vi "Save AO.vi"(8 "error in (no error)":errorcluster, 11 "Generator in":refnum<class "Generator.lvclass">) -> (0 "error out":errorcluster, 3 "Generator out":refnum<class "Generator.lvclass">)   [LabVIEW 2019, in "Generator.lvclass"]
uses:
  Generator.lvclass
  Generator.lvclass/Generator.ctl
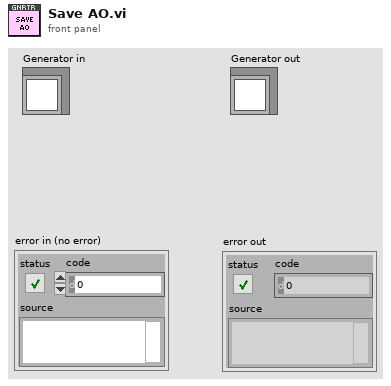
[diagram p1: front panel]
types:
  T1 = typedef "Generator.lvclass/AO.Channel--Cluster--Array.ctl" = T2[]
  T2 = typedef "Generator.lvclass/AO.Channel--Cluster.ctl" = cluster{"Enable?":bool, "Channel":i32, "Amplitude":dbl, "Offset":dbl, "Frequency":dbl, "Phase":dbl, "Function":T3, "Sweeping?":bool, "Limit AC?":bool, "Limit DC?":bool, "Duty Cycle?":bool, "Duty Cycle":dbl}
  T3 = typedef "Generator.lvclass/AO.Channel.Function--Enum.ctl" = enum16{"sine", "square", "triangle", "saw"}
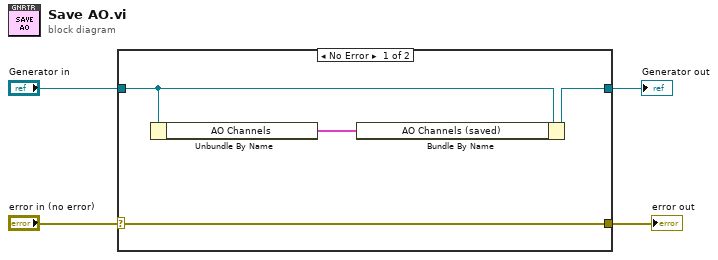
[diagram p0: block diagram]
diagram:
  n1 = case shown="No Error" "error in (no error)" {
    selector: "error in (no error)" -> [w5 w9]
    tunnel: "Generator in" -> [w7 w10]
    tunnel: [w6 w10] -> w3
    tunnel: [w5 w9] -> w1
    frame No Error {
      n2 = Unbundle By Name(w7) -> ("AO Channels"=w8:T1)
      n3 = Bundle By Name(cluster=w7, "AO Channels (saved)"=w8) -> (w6:refnum<class "Generator.lvclass">)
    }
    frame Error {
    }
  }
  "Generator out" <- w3
  "error out" <- w1
